vi "UN_PSWRD.vi"() -> ()   [LabVIEW 2020]
panel:
  in  "PASSWORD":string
  in  "USERNAME":string
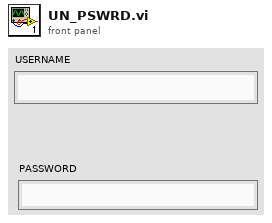
[diagram p1: front panel]
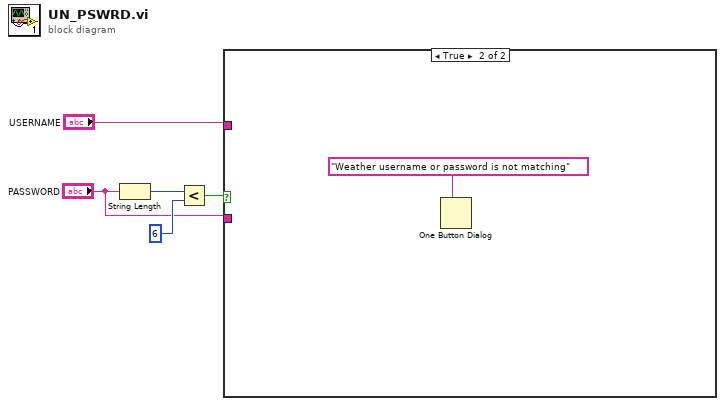
[diagram p0: block diagram]
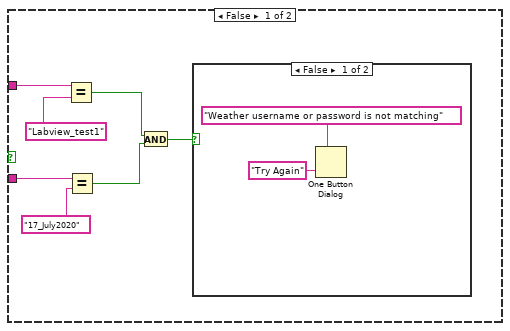
[diagram p2: hidden frame]
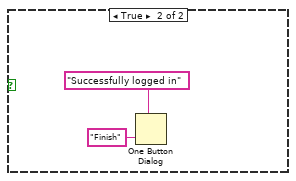
[diagram p3: hidden frame]
diagram:
  n1 = String Length(string="PASSWORD") -> (length=w5:i32)
  n2 = Less?(x=w5, y=6) -> (x < y?=w3:bool)
  n3 = case shown="True" w3 {
    tunnel: "USERNAME" -> [w12 _]
    tunnel: "PASSWORD" -> [w10 _]
    frame False {
      n4 = Equal?(x=w12, y="Labview_test1") -> (x = y?=w8:bool)
      n5 = Equal?(x=w10, y="17_July2020") -> (x = y?=w7:bool)
      n6 = And(x=w8, y=w7) -> (x .and. y?=w6:bool)
      n7 = case shown="False" w6 {
        frame False {
          n8 = One Button Dialog(message="Weather username or password is not matching", button name ("OK")="Try Again") -> ()  [unwired: 1 out]
        }
        frame True {
          n9 = One Button Dialog(message="Successfully logged in", button name ("OK")="Finish") -> ()  [unwired: 1 out]
        }
      }
    }
    frame True {
      n10 = One Button Dialog(message="Weather username or password is not matching") -> ()  [unwired: 1 in, 1 out]
    }
  }
